vi "setbitrate.vi"(8 "error in (no error)":errorcluster, 9 "NetworkID":i8(ring) items=["NETID_DEVICE"=0, "NETID_HSCAN"=1, "NETID_MSCAN"=2, "NETID_SWCAN"=3, "NETID_LSFTCAN"=4, "NETID_FORDSCP"=5, "NETID_J1708"=6, "NETID_AUX"=7, "NETID_JVPW"=8, "NETID_ISO_LIN"=9, "NETID_ISOPIC"=10, "NETID_MAIN51"=11, "NETID_SCI"=13, "NETID_ISO2"=14, "NETID_FIRE_HSCAN1"=41, "NETID_FIRE_HSCAN2"=42, "NETID_FIRE_MSCAN1"=43, "NETID_FIRE_MSCAN2_HSCAN3"=44, "NETID_FIRE_SWCAN"=45, "NETID_FIRE_LSFT"=46, "NETID_FIRE_LIN1"=47, "NETID_FIRE_LIN2"=48, "NETID_FIRE_LIN3"=49, "NETID_FIRE_LIN4"=50], 10 "BitRate":i32, 11 "hObject":i32) -> (0 "error out":errorcluster, 3 "hObject Out":i32)   [LabVIEW 2018]
doc: "this vi sets the bitrate of the device\n\n12/21/2010 1.0.0 jyg\n- initial release"
uses:
  icsneo40.dll
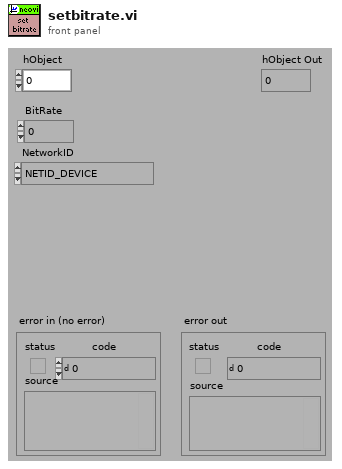
[diagram p1: front panel]
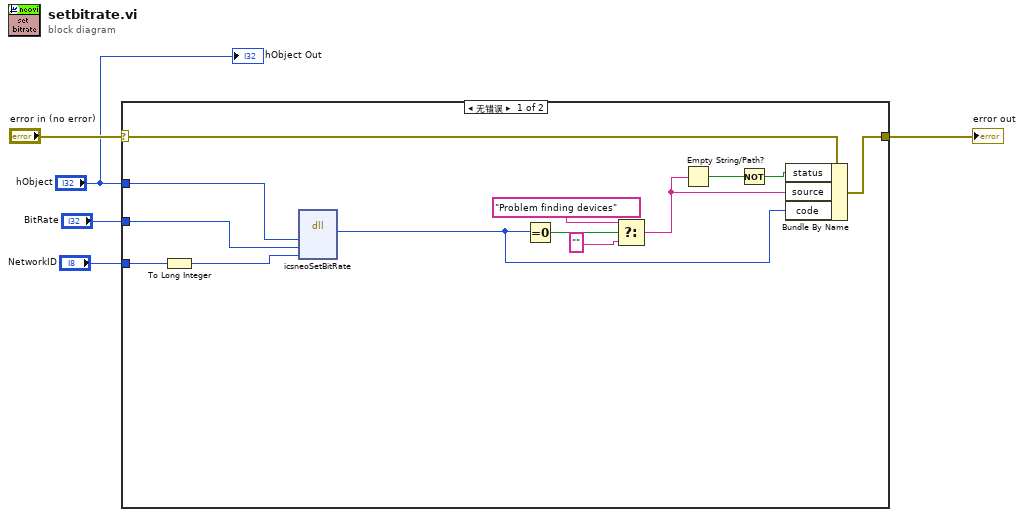
[diagram p0: block diagram]
diagram:
  n1 = case shown="无错误" "error in (no error)" {
    selector: "error in (no error)" -> [w14 w19]
    tunnel: "hObject" -> [w9 _]
    tunnel: [w15 w19] -> w5
    tunnel: "BitRate" -> [w8 _]
    tunnel: "NetworkID" -> [w7 _]
    frame No Error {
      n2 = To Long Integer(number=w7) -> (32bit integer=w6:i32)
      n3 = dll-call lib="icsneo40.dll" fn="icsneoSetBitRate"("hObject"=w9, "BitRate"=w8, "NetworkID"=w6) -> ("return type"=w13:i32)  [unwired: 6 in, 2 out]
      n4 = Equal To 0?(x=w13) -> (x = 0?=w12:bool)
      n5 = Select(t="Problem finding devices", s=w12, f="") -> (s? t:f=w11:string)
      n6 = Empty String/Path?(string/path=w11) -> (empty?=w17:bool)
      n7 = Not(x=w17) -> (.not. x?=w16:bool)
      n8 = Bundle By Name(cluster=w14, "status"=w16, "source"=w11, "code"=w13) -> (w15:errorcluster)
    }
    frame Error {
    }
  }
  "error out" <- w5
  "hObject Out" <- "hObject"
